vi "Get_Moving_Average.vi"(0 "Generated_Data_Preview":dbl[](array[numeric]), 5 "Moving_Average":i32) -> (4 "Numeric":dbl)   [LabVIEW 2021]
doc: "This VI Gives out the moving average value, calculated from the data given in"
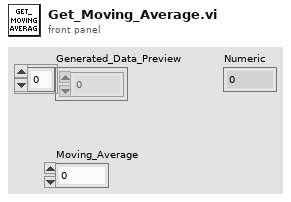
[diagram p1: front panel]
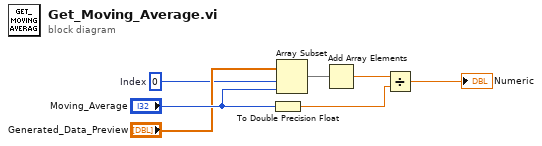
[diagram p0: block diagram]
diagram:
  w1 = 0  # Index
  n1 = To Double Precision Float(number="Moving_Average") -> (double precision float=w6:dbl)
  n2 = Array Subset "Array Subset"(array="Generated_Data_Preview", index=w1, length="Moving_Average") -> (w2:dbl[])
  n3 = Add Array Elements(numeric array=w2) -> (sum=w5:dbl)
  n4 = Divide(x=w5, y=w6) -> (x/y=→"Numeric":dbl)
